vi "Create Class ObjectData DVR.vi"(8 "error in (no error)":errorcluster, 11 "Application in":refnum<class "Application.lvclass">) -> (0 "error out":errorcluster, 3 "Application out":refnum<class "Application.lvclass">)   [LabVIEW 2019, in "Application.lvclass"]
doc: "Developed by Kevin Thompson\nkevin@thompsonengineering.net\n\nCopyright 2018\nThompson Engineering, LLC"
uses:
  Application.lvclass
  DataTypes/ObjData--cluster.ctl
  DataTypes/Read Data--cluster.ctl
  DataTypes/Settings--cluster.ctl
  DataTypes/Dependency--cluster.ctl
  Common/DataTypes/TD Async CmdMsg EventData--cluster.ctl
  DataTypes/Public Events--cluster.ctl
  <vilib>/TELLC/Dynamic CVT API/TD Dynamic CVT DVR--ref.ctl
  Subsystems/Log_Engine/Log_Engine.lvclass
  Subsystems/DAQ_Engine/DAQ_Engine.lvclass
  Common/ErrorHandler/ErrorHandler.lvclass
  Subsystems/Main/Main.lvclass
  Subsystems/Config/Config.lvclass
  Common/DataTypes/RawChannelData--cluster.ctl
  Common/DataTypes/RawDAQData--cluster.ctl
  Common/DataTypes/RawDAQDataQRef--cluster.ctl
  Common/DataTypes/ChannelWaveforms--cluster.ctl
  Common/DataTypes/InverterWaveforms--cluster.ctl
  Common/DataTypes/InverterWaveforms--QRef.ctl
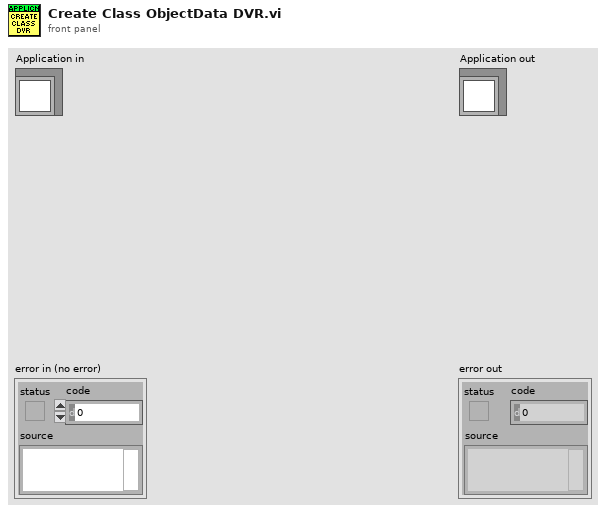
[diagram p1: front panel]
types:
  T1 = typedef "Application.lvclass/ObjData--cluster.ctl" = cluster{"Settings":T2, "Public Events":T3, "Dependency":T4, "ReadData-placeholder":T5, "VISA-placeholder":refnum<visa-resource-name>, "Subsys ClassRefs Dict":T6, "InverterWaveformsQ":T7, "RawDaqDataQ":T8}
  T2 = typedef "Application.lvclass/Settings--cluster.ctl" = cluster{"Simulation":bool}
  T3 = typedef "Application.lvclass/Public Events--cluster.ctl" = cluster{"Application.AsyncCmd Event":refnum<user-event>, "Application.AsyncMsg Event":refnum<user-event>, "stop process":refnum<user-event>}
  T4 = typedef "Application.lvclass/Dependency--cluster.ctl" = cluster{"Config":refnum<class "Config.lvclass">, "Main":refnum<class "Main.lvclass">, "ErrorHandler":refnum<class "ErrorHandler.lvclass">, "DAQ_Engine":refnum<class "DAQ_Engine.lvclass">, "Log_Engine":refnum<class "Log_Engine.lvclass">}
  T5 = typedef "Application.lvclass/Read Data--cluster.ctl" = cluster{"Data":dbl}
  T6 = typedef "TD Dynamic CVT DVR--ref.ctl" = refnum<data-value>
  T7 = typedef "InverterWaveforms--QRef.ctl" = refnum<queue>
  T8 = typedef "RawDAQDataQRef--cluster.ctl" = refnum<queue>
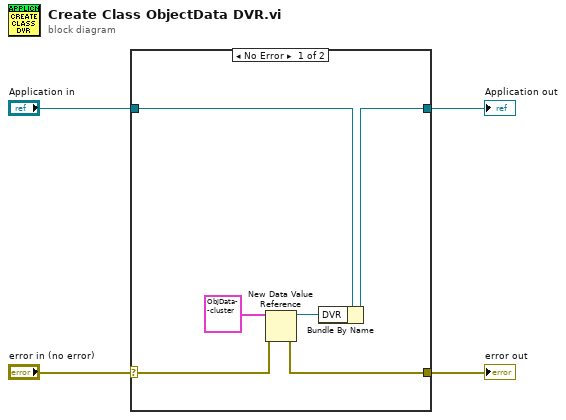
[diagram p0: block diagram]
diagram:
  n1 = case shown="No Error" "error in (no error)" {
    selector: "error in (no error)" -> [w9 w12]
    tunnel: [w8 w12] -> w3
    tunnel: [w6 w11] -> w1
    tunnel: "Application in" -> [w7 w11]
    frame No Error {
      n2 = New Data Value Reference(data value=T1 {"Settings"={"Simulation"=FALSE}, "Public Events"={"Application.AsyncCmd Event"=refnum, "Application.AsyncMsg Event"=refnum, "stop process"=refnum}, "Dependency"={"Config"=refnum, "Main"=refnum, "ErrorHandler"=refnum, "DAQ_Engine"=refnum, "Log_Engine"=refnum}, "ReadData-placeholder"={"Data"=0.0}, "VISA-placeholder"="", "Subsys ClassRefs Dict"=refnum, "InverterWaveformsQ"=refnum, "RawDaqDataQ"=refnum} ("ObjData"), error in=w9) -> (data value reference=w10:refnum<data-value>, error out=w8:errorcluster)
      n3 = Bundle By Name(cluster=w7, "DVR"=w10) -> (w6:refnum<class "Application.lvclass">)
    }
    frame Error {
    }
  }
  "error out" <- w3
  "Application out" <- w1
